vi "Test UI-Bus U8 Vars.vi"() -> ()   [LabVIEW 2021]
uses:
  Source/UI-Bus/UI-Bus.lvclass
  C:/Program Files (x86)/National Instruments/LabVIEW 2021/vi.lib/TSA/Omni-Bus/Omni-Bus/Bus Access/Bus_Access.lvclass
  <vilib>/TSA/Omni-Bus/Omni-Bus/Omni_Bus.lvclass
  <vilib>/TSA/Omni-Bus/Omni-Bus/Support/Broad Types.ctl
  <vilib>/Utility/Data Type/Type Definitions/Data Type.ctl
  <vilib>/TSA/Abstract Data Classes/Abs_Types/Type/Abs_Type.lvclass/Abs_Type.ctl
  <vilib>/TSA/Omni-Bus/Omni-Bus/Omni_Bus.lvclass/Omni_Bus.ctl
  <vilib>/TSA/Omni-Bus/Omni-Bus/Support/Read/Read Multi U8.vi
  <vilib>/TSA/Omni-Bus/Omni-Bus/Support/Write/Write U8.vi
  <vilib>/TSA/Omni-Bus/Omni-Bus/Support/Get/Get Multi U8.vi
  <vilib>/TSA/Omni-Bus/Omni-Bus/Support/FindVar.vi
  <vilib>/TSA/Omni-Bus/Omni-Bus/Support/FindMultiVar.vi
  <vilib>/Utility/error.llb/Clear Errors.vi
  <vilib>/TSA/Omni-Bus/Omni-Bus/Properties/Read Var Map.vi
  <vilib>/TSA/Abstract Data Classes/Abs_Types/Type/Properties/Read Tag.vi
  <vilib>/TSA/Abstract Data Classes/Abs_Types/U8 Integer/Abs_U8 Integer.lvclass
  C:/Program Files (x86)/National Instruments/LabVIEW 2021/vi.lib/TSA/Abstract Data Classes/Abs_Types/Type/Abs_Type.lvclass
  <vilib>/TSA/Abstract Data Classes/Abs_Types/Value/Abs_Value.lvclass
  <vilib>/TSA/Omni-Bus/Omni-Bus/Support/Check For Read Only Error.vi
  <vilib>/TSA/Omni-Bus/Omni-Bus/Support/Incorrect Tag String Error.vi
  <vilib>/TSA/Abstract Data Classes/Abs_Types/Type/Abs_Type.lvclass
  <vilib>/Utility/Data Type/NI_Data Type.lvlib
panel:
  out "Thermometer":u8(slide) scale=0.0..100.0
  out "Tank":u8(slide) scale=0.0..10.0
  out "Gauge":u8(knob) scale=0.0..10.0
  out "Meter":u8(knob) scale=0.0..10.0
  in  "Dial":u8(knob) scale=0.0..10.0
  in  "Knob":u8(knob) scale=0.0..10.0
  out "Slide 9":u8(slide) scale=0.0..100.0
  out "Slide 8":u8(slide) scale=0.0..100.0
  in  "Slide 7":u8(slide) scale=0.0..10.0
  in  "Slide 6":u8(slide) scale=0.0..10.0
  out "Slide 5":u8(slide) scale=0.0..100.0
  out "Slide 4":u8(slide) scale=0.0..100.0
  out "Slide 3":u8(slide) scale=0.0..100.0
  in  "Slide 2":u8(slide) scale=0.0..10.0
  in  "Slide":u8(slide) scale=0.0..10.0
  out "Numeric 3":u8
  in  "Numeric 2":u8
  in  "#Numeric":u8
  out "U8's":u8[](array[numeric])
  in  "Tag List":string(combo)
  out "error":errorcluster
  in  "stop":bool
  out "Tags":string[](array[string])
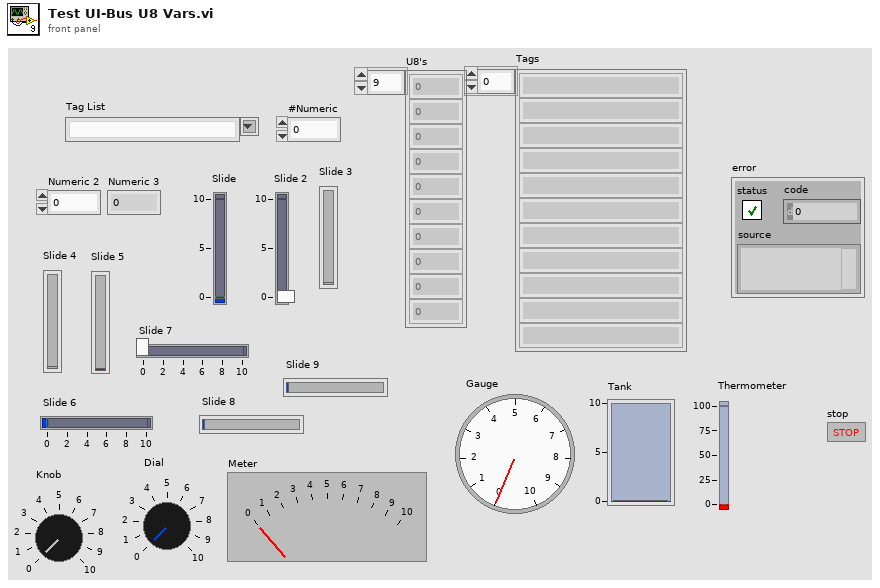
[diagram p1: front panel]
types:
  T1 = typedef "NI_Data Type.lvlib/Data Type.ctl" = enum8{"Invalid Type", "Void", "I8", "I16", "I32", "I64", "U8", "U16", "U32", "U64", "Single Float", "Double Float", "Extended Float", "Single Complex", "Double Complex", "Extended Complex", "Enum U8", "Enum U16", "Enum U32", "Enum U64", "Single Float With Unit", "Double Float With Unit", "Extended Float With Unit", "Single Complex with Unit", "Double Complex with Unit", "Extended Complex with Unit", "Boolean", "String", "Path", "Picture", "Tag", "Array", "Cluster", "Variant", "LV Variant", "Waveform", "Timestamp", "Digital Waveform", "Digital Data", "ExpressData", "Refnum", "External Data", "VI", "Poly VI", "LabVIEW Class Instance", "Fixed Point", "Set Collection", "Map Collection"}
  T2 = typedef "Omni_Bus.lvclass/Broad Types.ctl" = enum16{"All Tags", "NI Specific Type", "Boolean", "String", "Numeric", "Float", "Integer", "Collection", "All Value Types", "Non Value Types"}
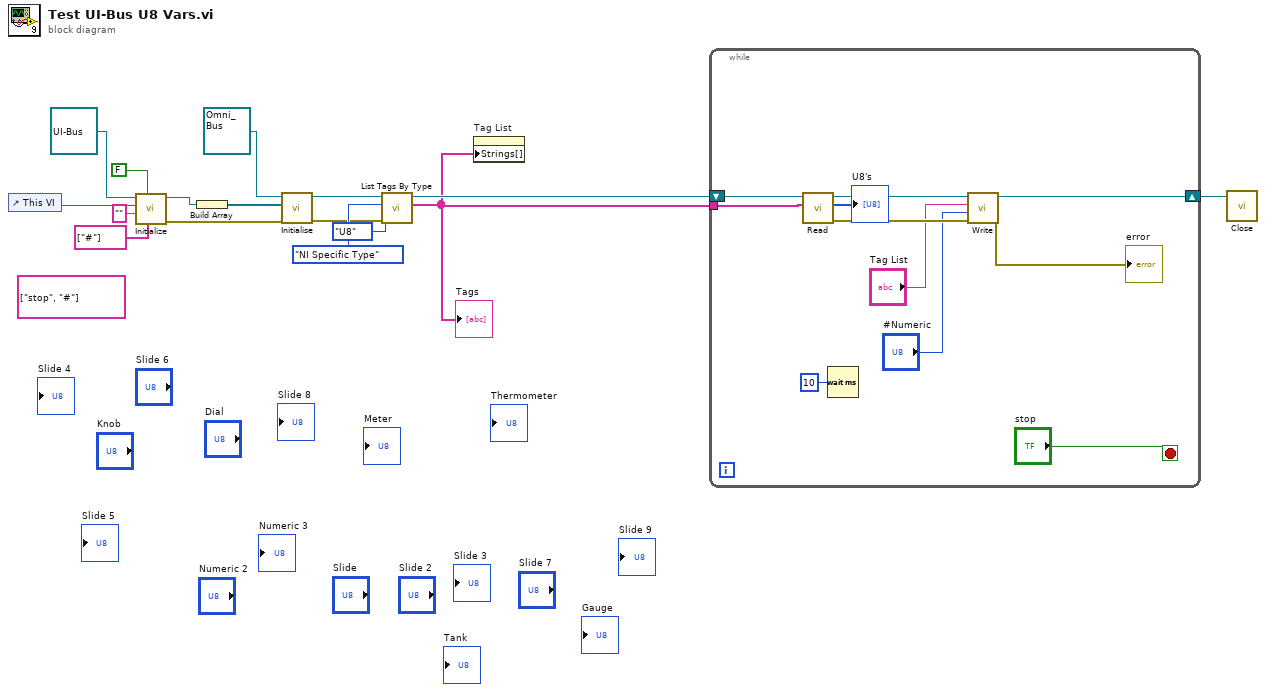
[diagram p0: block diagram]
diagram:
  (unwired) string[] ["stop", "#"] ("Label Black List")
  n1 = control-ref of="This VI"() -> (w15:refnum<vi>)
  n2 = call "Initialize.vi"("Label Match White List"=string[] ["#"], "Tab Label in Tag"=FALSE, "Tag Root"="", "VI Refnum"=w15, "UI-Bus in"=refnum<class "UI-Bus.lvclass"> refnum) -> ("error out"=w11:errorcluster, "UI-Bus out"=w13:refnum<class "UI-Bus.lvclass">)  [unwired: 5 in]
  n3 = Build Array(w13) -> (w12:refnum<class "UI-Bus.lvclass">[])
  n4 = call-dynamic "Initialise.vi"("error in (no error)"=w11, "Bus Access"=w12, "Var Bus in"=refnum<class "Omni_Bus.lvclass"> refnum) -> ("error out"=w4:errorcluster, "Var Bus out"=w5:refnum<class "Omni_Bus.lvclass">)  [unwired: 7 in]
  n5 = call <vilib>:"List Tags By Type.vi"("error in (no error)"=w4, "NI Specific Type"=Data_Type."U8", "Broad Types"=Broad_Types."NI Specific Type", "Var Bus in"=w5) -> ("Tags"=w3:string[], "Var Bus out"=w9:refnum<class "Omni_Bus.lvclass">)  [unwired: 4 in, 2 out]
  "Tags" <- w3
  n6 = property on="Tag List" class="CmbBox"("Strings[]"=w3) -> ()  [unwired: 2 in, 2 out]
  n7 = while {
    tunnel: w3 -> [w27]
    shift-right: [w21] -> w8
    shift-left: w9 -> [w26]
    stop <- "stop" stop-if-true
    n8 = call-poly <vilib>:"Read.vi"("Tag"=w27, "Var Bus in"=w26) -> ("error out"=w22:errorcluster, "U8's"=→"U8's":u8[], "Var Bus out"=w23:refnum<class "Omni_Bus.lvclass">)  [unwired: 7 in]
    n9 = Wait (ms)(milliseconds to wait=u32 10) -> ()  [unwired: 1 out]
    n10 = call-poly <vilib>:"Write.vi"("error in (no error)"=w22, "Numeric"="#Numeric", "Tag"="Tag List", "Omni_Bus in"=w23) -> ("error out"=→"error":errorcluster, "Omni_Bus out"=w21:refnum<class "Omni_Bus.lvclass">)  [unwired: 6 in]
  }
  n11 = call-dynamic "Close.vi"("Data in"=w8) -> ()  [unwired: 9 in, 2 out]
